vi "Run.vi"(7 "Team Index":i32, 8 "Column":i32, 9 "Row":i32, 10 "View":i32[](array[numeric]) caption="View (Team Index, -1: empty)", 11 "Runner in":refnum<class "Formation.lvclass">) -> (0 "Replicated":refnum<class "Square.lvclass">, 1 "Direction":T1, 2 "Action":T2, 3 "Runner out":refnum<class "Formation.lvclass">)   [LabVIEW 2015, in "Formation.lvclass"]
uses:
  Formation.lvclass
  Type Defs/Action Enum.ctl
  Type Defs/Direction Enum.ctl
  Square/Square.lvclass
  Formation.lvclass/Formation.ctl
  DVR Data Cluster.ctl
  Board Cluster.ctl
  SubVIs/Read-Only Globals.vi
  SubVIs/Globals (private).vi
  Common/Find Enemy.vi
  Common/Reverse Direction.vi
  Type Defs/SB Type Defs.lvlib
  Common/Common.lvlib
panel:
  # "NW\nN\nNE\nE\nSE\nS\nSW\nW"
  # "NOTICE - YOU MUST NOT REMOVE THIS NOTICE. PER THE FOLLOWING LICENSE, YOU MAY REPRODUCE THIS SOFTWARE PROVIDED YOU FOLLOW THE TERMS\nOF THE LICENSE.\n\n---BEGIN BSD LICENSE (http://opensource.org/licenses/BSD-2-Clause)---\nCopyright (c) 2015, Endigit, Inc. <robert@endigit.com>\nAll rights reserved.\n\nRedistribution and use in source and binary forms, with or without modification, are permitted provided that the following conditions are met:\n\n1. Redistributions of source code must retain the above copyright notice, this list of conditions and the following disclaimer.\n\n2. Redistributions in binary form must reproduce the above copyright notice, this list of conditions and the following disclaimer in the documentation and/or other \nmaterials provided with the distribution.\n\nTHIS SOFTWARE IS PROVIDED BY THE COPYRIGHT HOLDERS AND CONTRIBUTORS \"AS IS\" AND ANY EXPRESS OR IMPLIED WARRANTIES, INCLUDING, BUT NOT \nLIMITED TO, THE IMPLIED WARRANTIES OF MERCHANTABILITY AND FITNESS FOR A PARTICULAR PURPOSE ARE DISCLAIMED. IN NO EVENT SHALL THE COPYRIGHT \nHOLDER OR CONTRIBUTORS BE LIABLE FOR ANY DIRECT, INDIRECT, INCIDENTAL, SPECIAL, EXEMPLARY, OR CONSEQUENTIAL DAMAGES (INCLUDING, BUT NOT \nLIMITED TO, PROCUREMENT OF SUBSTITUTE GOODS OR SERVICES; LOSS OF USE, DATA, OR PROFITS; OR BUSINESS INTERRUPTION) HOWEVER CAUSED AND ON \nANY THEORY OF LIABILITY, WHETHER IN CONTRACT, STRICT LIABILITY, OR TORT (INCLUDING NEGLIGENCE OR OTHERWISE) ARISING IN ANY WAY OUT OF THE USE \nOF THIS SOFTWARE, EVEN IF ADVISED OF THE POSSIBILITY OF SUCH DAMAGE.\n---END BSD LICENSE---"
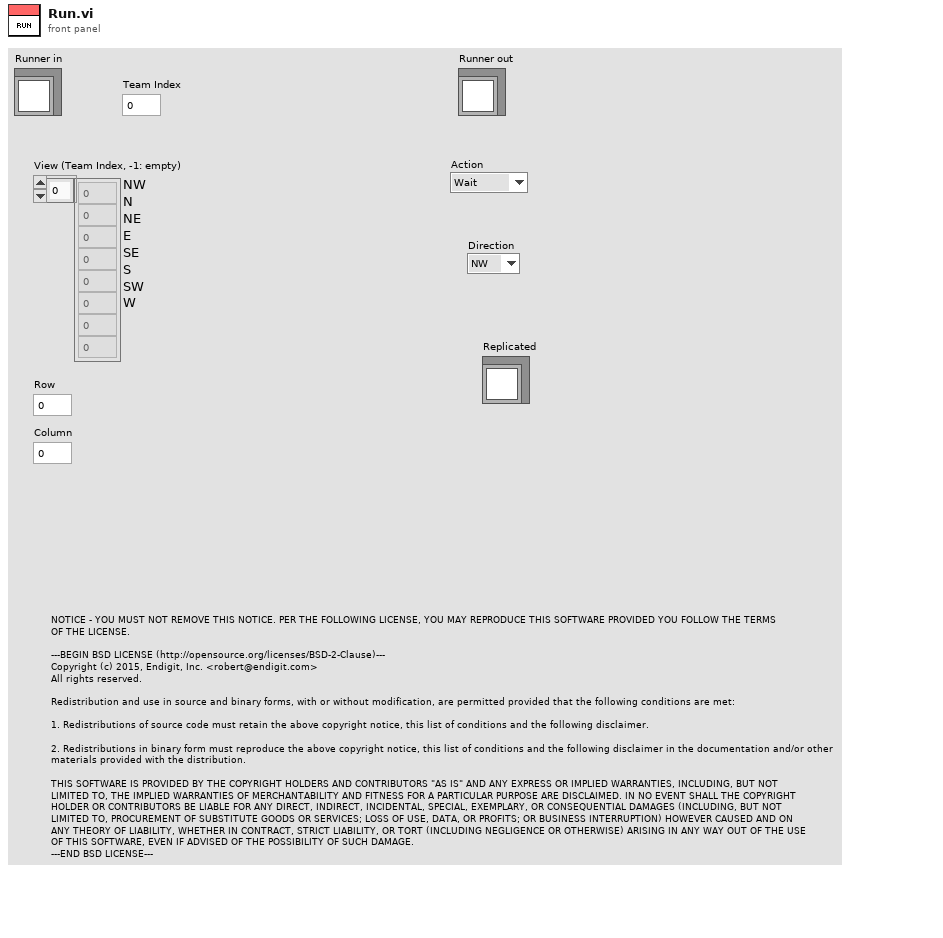
[diagram p1: front panel]
types:
  T1 = typedef "SB Type Defs.lvlib/Direction Enum.ctl" = enum16{"NW", "N", "NE", "E", "SE", "S", "SW", "W"}
  T2 = typedef "SB Type Defs.lvlib/Action Enum.ctl" = enum16{"Wait", "Move", "Attack", "Replicate"}
  T3 = cluster{"Options":cluster{"X":i8, "Y":i8, "SignMatch":i8, "Action":T2, "Direction":T1, "Unit Idx":u8}[]}[]
  T4 = typedef "Formation.lvclass/DVR Data Cluster.ctl" = cluster{"Moved[Id]":i64, "UnitRound":i32, "Direction":T1, "FormIdx":i32, "LastSpawn":i32, "Spawning?":bool, "SpawnDist":i32}
  T5 = cluster{"Options":cluster{"X":i8, "Y":i8, "SignMatch":i8, "Action":T2, "Direction":T1, "Unit Idx":u8}[]}
  T6 = cluster{"X":i8, "Y":i8, "SignMatch":i8, "Action":T2, "Direction":T1, "Unit Idx":u8}[]
  T7 = typedef "Formation.lvclass/Board Cluster.ctl" = cluster{"Board S":i32, "Pos[Idx]":cluster{"X":i32, "Y":i32}[], "Round[Idx]":i32[]}
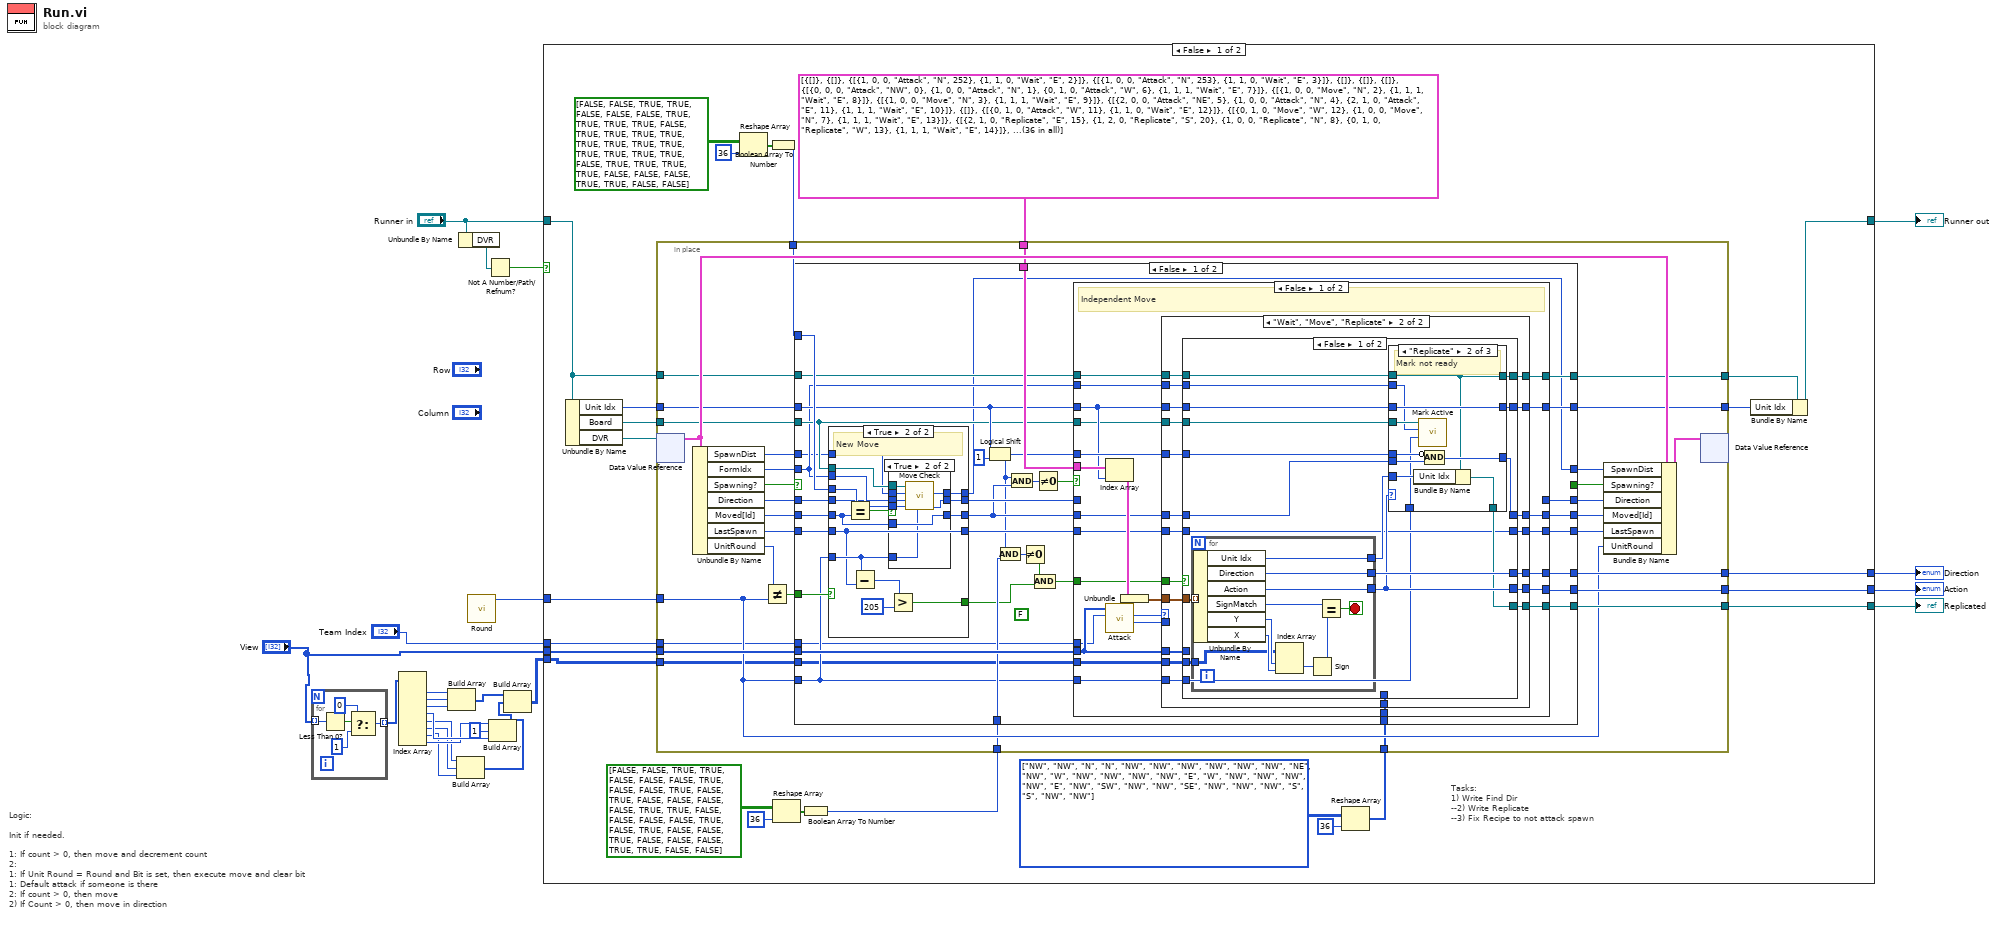
[diagram p0: block diagram]
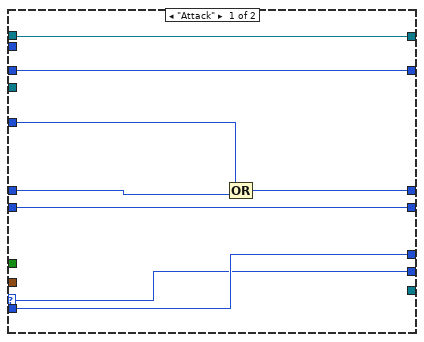
[diagram p2: hidden frame]
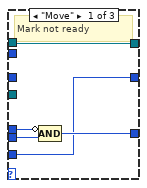
[diagram p3: hidden frame]
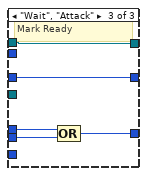
[diagram p4: hidden frame]
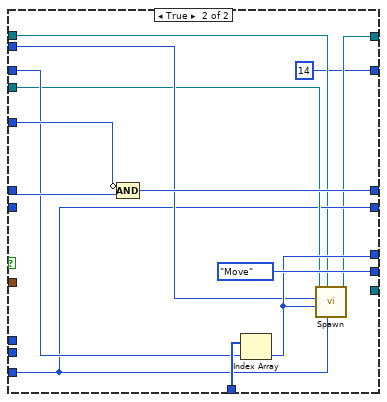
[diagram p5: hidden frame]
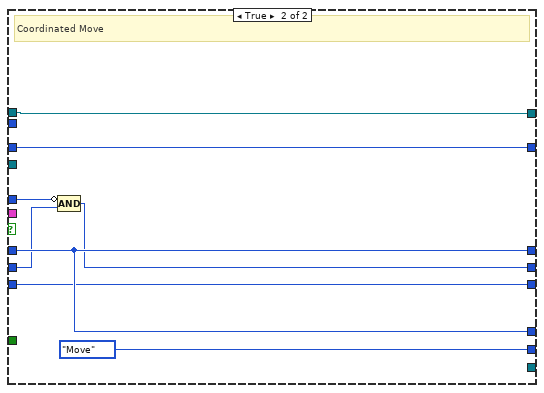
[diagram p6: hidden frame]
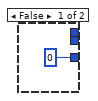
[diagram p8: hidden frame]
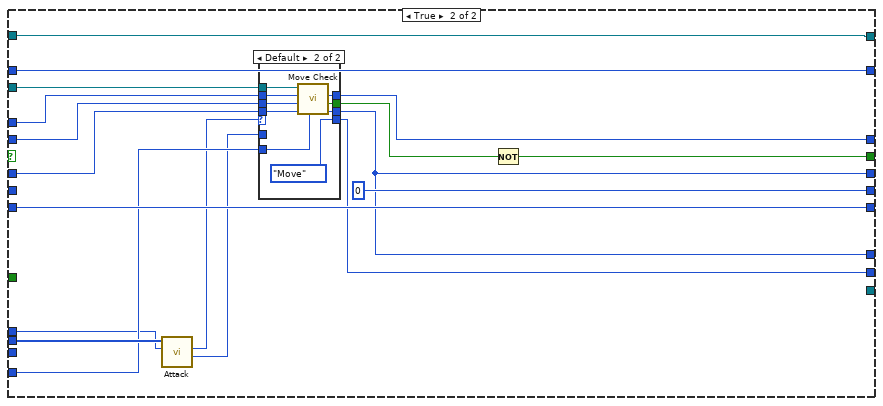
[diagram p9: hidden frame]
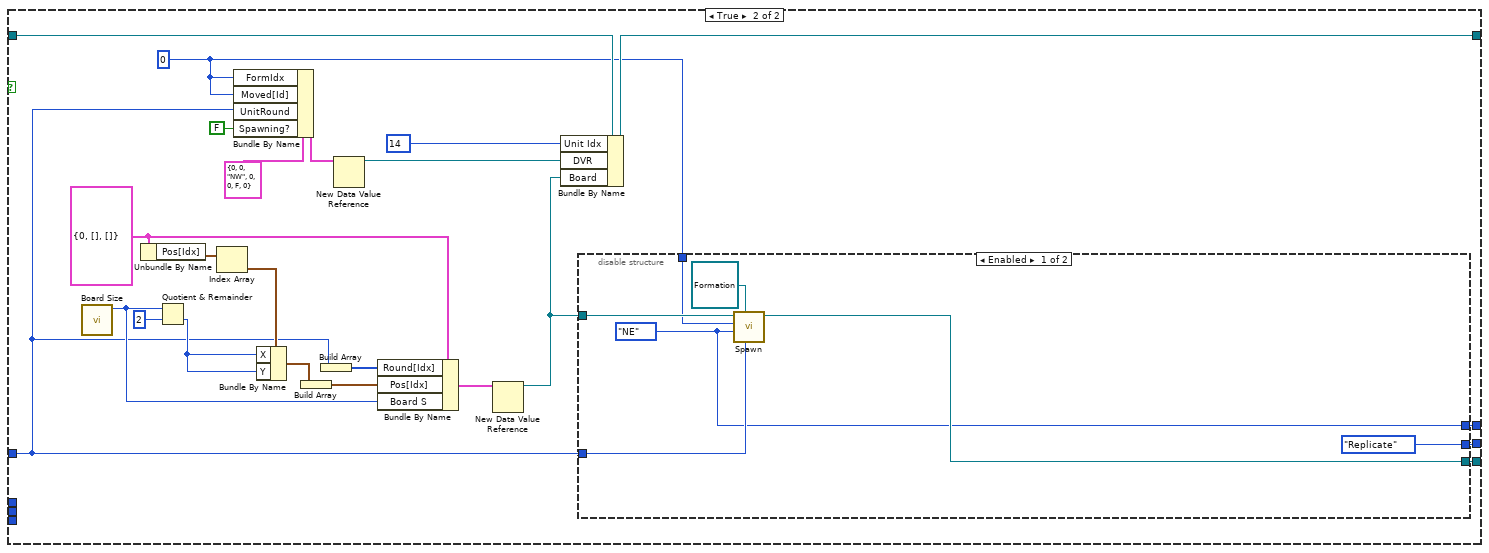
[diagram p11: hidden frame]
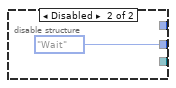
[diagram p12: hidden frame]
diagram:
  # "Logic:\n\nInit if needed.\n\n1: If count > 0, then move and decrement count\n2: \n1: If Unit Round = Round and Bit is set, then execute move and clear bit\n1: Default attack if someone is there\n2: If count > 0, then move\n2) If Count > 0, then move in direction"
  n1 = for {
    tunnel: "View" -> [w29] mode=indexing
    tunnel: [w26] -> w5 mode=indexing
    n2 = Less Than 0?(x=w29) -> (x < 0?=w28:bool)
    n3 = Select(t=0, s=w28, f=1) -> (s? t:f=w26:i32)
  }
  n4 = Index Array(array=w5) -> (element #1=w15:i32, element #2=w14:i32, element #3=w13:i32, element #4=w12:i32, element #5=w9:i32, element #6=w8:i32, element #7=w7:i32, element #8=w11:i32)  [unwired: 8 in]
  n5 = Build Array(w15, w14, w13) -> (w4:i32[])
  n6 = Build Array(w9, w8, w7) -> (w2:i32[])
  n7 = Unbundle By Name("Runner in") -> ("DVR"=w24:refnum<data-value>)
  n8 = call "Round.vi"() -> ("Round"=w23:i32)  [unwired: 11 in]
  n9 = Not A Number/Path/Refnum?(number/path/refnum=w24) -> (NaN/Path/Refnum?=w18:bool)
  n10 = Build Array(w11, 1 ("element"), w12) -> (w3:i32[])
  n11 = Build Array(w4, w3, w2) -> (w1:i32[][])
  n12 = case shown="False" w18 {
    tunnel: w23 -> [w52 w305]
    tunnel: "View" -> [w51 _]
    tunnel: [w50 w304] -> w22
    tunnel: [w49 w319] -> w21
    tunnel: [w44 w321] -> w20
    tunnel: "Runner in" -> [w42 w325]
    tunnel: [w41 w307] -> w19
    tunnel: "Team Index" -> [w31 _]
    tunnel: w1 -> [w30 _]
    frame False {
      w36 = T1[][] [[enum."NW", enum."NW", enum."N", enum."N", enum."NW", enum."NW"], [enum."NW", enum."NW", enum."NW", enum."NW", enum."NE", enum."NW"], [enum."W", enum."NW", enum."NW", enum."NW", enum."NW", enum."E"], [enum."W", enum."NW", enum."NW", enum."NW", enum."NW", enum."E"], [enum."NW", enum."SW", enum."NW", enum."NW", enum."SE", enum."NW"], [enum."NW", enum."NW", enum."S", enum."S", enum."NW", enum."NW"]] items=["NW", "N", "NE", "E", "SE", "S", "SW", "W"]
      # "Tasks: \n1) Write Find Dir\n--2) Write Replicate\n--3) Fix Recipe to not attack spawn"
      n13 = Unbundle By Name(w42) -> ("Unit Idx"=w54:u16, "Board"=w55:refnum<data-value>, "DVR"=w53:refnum<data-value>)
      n14 = Reshape Array(bool[][] [[FALSE, FALSE, TRUE, TRUE, FALSE, FALSE], [FALSE, TRUE, TRUE, TRUE, TRUE, FALSE], [TRUE, TRUE, TRUE, TRUE, TRUE, TRUE], [TRUE, TRUE, TRUE, TRUE, TRUE, TRUE], [FALSE, TRUE, TRUE, TRUE, TRUE, FALSE], [FALSE, FALSE, TRUE, TRUE, FALSE, FALSE]], 36 ("dimension size")) -> (w46:bool[])
      n15 = Boolean Array To Number(Boolean array=w46) -> (number=w45:i64)
      n16 = Reshape Array(bool[][] [[FALSE, FALSE, TRUE, TRUE, FALSE, FALSE], [FALSE, TRUE, FALSE, FALSE, TRUE, FALSE], [TRUE, FALSE, FALSE, FALSE, FALSE, TRUE], [TRUE, FALSE, FALSE, FALSE, FALSE, TRUE], [FALSE, TRUE, FALSE, FALSE, TRUE, FALSE], [FALSE, FALSE, TRUE, TRUE, FALSE, FALSE]], 36 ("dimension size")) -> (w38:bool[])
      n17 = Boolean Array To Number(Boolean array=w38) -> (number=w37:i64)
      n18 = Reshape Array(w36, 36 ("dimension size")) -> (w34:T1[])
      n19 = in-place {
        in-place-border: w54 -> [w75]
        in-place-border: w55 -> [w69]
        in-place-border: w51 -> [w73]
        in-place-border: w52 -> [w67]
        in-place-border: [w80] -> w50
        in-place-border: [w79] -> w49
        in-place-border: w45 -> [w77]
        in-place-border: T3 [{"Options"=[]}, {"Options"=[]}, {"Options"=[{"X"=1, "Y"=0, "SignMatch"=0, "Action"=enum."Attack", "Direction"=enum."N", "Unit Idx"=252}, {"X"=1, "Y"=1, "SignMatch"=0, "Action"=enum."Wait", "Direction"=enum."E", "Unit Idx"=2}]}, {"Options"=[{"X"=1, "Y"=0, "SignMatch"=0, "Action"=enum."Attack", "Direction"=enum."N", "Unit Idx"=253}, {"X"=1, "Y"=1, "SignMatch"=0, "Action"=enum."Wait", "Direction"=enum."E", "Unit Idx"=3}]}, {"Options"=[]}, {"Options"=[]}, {"Options"=[]}, {"Options"=[{"X"=0, "Y"=0, "SignMatch"=0, "Action"=enum."Attack", "Direction"=enum."NW", "Unit Idx"=0}, {"X"=1, "Y"=0, "SignMatch"=0, "Action"=enum."Attack", "Direction"=enum."N", "Unit Idx"=1}, {"X"=0, "Y"=1, "SignMatch"=0, "Action"=enum."Attack", "Direction"=enum."W", "Unit Idx"=6}, {"X"=1, "Y"=1, "SignMatch"=1, "Action"=enum."Wait", "Direction"=enum."E", "Unit Idx"=7}]}, {"Options"=[{"X"=1, "Y"=0, "SignMatch"=0, "Action"=enum."Move", "Direction"=enum."N", "Unit Idx"=2}, {"X"=1, "Y"=1, "SignMatch"=1, "Action"=enum."Wait", "Direction"=enum."E", "Unit Idx"=8}]}, {"Options"=[{"X"=1, "Y"=0, "SignMatch"=0, "Action"=enum."Move", "Direction"=enum."N", "Unit Idx"=3}, {"X"=1, "Y"=1, "SignMatch"=1, "Action"=enum."Wait", "Direction"=enum."E", "Unit Idx"=9}]}, {"Options"=[{"X"=2, "Y"=0, "SignMatch"=0, "Action"=enum."Attack", "Direction"=enum."NE", "Unit Idx"=5}, {"X"=1, "Y"=0, "SignMatch"=0, "Action"=enum."Attack", "Direction"=enum."N", "Unit Idx"=4}, {"X"=2, "Y"=1, "SignMatch"=0, "Action"=enum."Attack", "Direction"=enum."E", "Unit Idx"=11}, {"X"=1, "Y"=1, "SignMatch"=1, "Action"=enum."Wait", "Direction"=enum."E", "Unit Idx"=10}]}, {"Options"=[]}, {"Options"=[{"X"=0, "Y"=1, "SignMatch"=0, "Action"=enum."Attack", "Direction"=enum."W", "Unit Idx"=11}, {"X"=1, "Y"=1, "SignMatch"=0, "Action"=enum."Wait", "Direction"=enum."E", "Unit Idx"=12}]}, {"Options"=[{"X"=0, "Y"=1, "SignMatch"=0, "Action"=enum."Move", "Direction"=enum."W", "Unit Idx"=12}, {"X"=1, "Y"=0, "SignMatch"=0, "Action"=enum."Move", "Direction"=enum."N", "Unit Idx"=7}, {"X"=1, "Y"=1, "SignMatch"=1, "Action"=enum."Wait", "Direction"=enum."E", "Unit Idx"=13}]}, {"Options"=[{"X"=2, "Y"=1, "SignMatch"=0, "Action"=enum."Replicate", "Direction"=enum."E", "Unit Idx"=15}, {"X"=1, "Y"=2, "SignMatch"=0, "Action"=enum."Replicate", "Direction"=enum."S", "Unit Idx"=20}, {"X"=1, "Y"=0, "SignMatch"=0, "Action"=enum."Replicate", "Direction"=enum."N", "Unit Idx"=8}, {"X"=0, "Y"=1, "SignMatch"=0, "Action"=enum."Replicate", "Direction"=enum."W", "Unit Idx"=13}, {"X"=1, "Y"=1, "SignMatch"=1, "Action"=enum."Wait", "Direction"=enum."E", "Unit Idx"=14}]}, {"Options"=[{"X"=1, "Y"=2, "SignMatch"=0, "Action"=enum."Replicate", "Direction"=enum."S", "Unit Idx"=21}, {"X"=1, "Y"=0, "SignMatch"=0, "Action"=enum."Replicate", "Direction"=enum."N", "Unit Idx"=9}, {"X"=2, "Y"=1, "SignMatch"=0, "Action"=enum."Replicate", "Direction"=enum."E", "Unit Idx"=16}, {"X"=1, "Y"=1, "SignMatch"=1, "Action"=enum."Wait", "Direction"=enum."E", "Unit Idx"=15}]}, {"Options"=[{"X"=2, "Y"=1, "SignMatch"=0, "Action"=enum."Move", "Direction"=enum."E", "Unit Idx"=17}, {"X"=1, "Y"=0, "SignMatch"=0, "Action"=enum."Move", "Direction"=enum."N", "Unit Idx"=10}, {"X"=1, "Y"=1, "SignMatch"=1, "Action"=enum."Wait", "Direction"=enum."E", "Unit Idx"=16}]}, {"Options"=[{"X"=2, "Y"=1, "SignMatch"=0, "Action"=enum."Attack", "Direction"=enum."E", "Unit Idx"=18}, {"X"=1, "Y"=1, "SignMatch"=0, "Action"=enum."Wait", "Direction"=enum."E", "Unit Idx"=17}]}, {"Options"=[{"X"=0, "Y"=1, "SignMatch"=0, "Action"=enum."Attack", "Direction"=enum."W", "Unit Idx"=17}, {"X"=1, "Y"=1, "SignMatch"=0, "Action"=enum."Wait", "Direction"=enum."E", "Unit Idx"=18}]}, {"Options"=[{"X"=0, "Y"=1, "SignMatch"=0, "Action"=enum."Move", "Direction"=enum."W", "Unit Idx"=18}, {"X"=1, "Y"=2, "SignMatch"=0, "Action"=enum."Move", "Direction"=enum."S", "Unit Idx"=25}, {"X"=1, "Y"=1, "SignMatch"=1, "Action"=enum."Wait", "Direction"=enum."E", "Unit Idx"=19}]}, {"Options"=[{"X"=1, "Y"=0, "SignMatch"=0, "Action"=enum."Replicate", "Direction"=enum."N", "Unit Idx"=14}, {"X"=1, "Y"=2, "SignMatch"=0, "Action"=enum."Replicate", "Direction"=enum."S", "Unit Idx"=26}, {"X"=0, "Y"=1, "SignMatch"=0, "Action"=enum."Replicate", "Direction"=enum."W", "Unit Idx"=19}, {"X"=1, "Y"=1, "SignMatch"=1, "Action"=enum."Wait", "Direction"=enum."E", "Unit Idx"=20}]}, {"Options"=[{"X"=1, "Y"=0, "SignMatch"=0, "Action"=enum."Replicate", "Direction"=enum."N", "Unit Idx"=15}, {"X"=1, "Y"=2, "SignMatch"=0, "Action"=enum."Replicate", "Direction"=enum."S", "Unit Idx"=27}, {"X"=2, "Y"=1, "SignMatch"=0, "Action"=enum."Replicate", "Direction"=enum."E", "Unit Idx"=22}, {"X"=1, "Y"=1, "SignMatch"=1, "Action"=enum."Wait", "Direction"=enum."E", "Unit Idx"=21}]}, {"Options"=[{"X"=2, "Y"=1, "SignMatch"=0, "Action"=enum."Move", "Direction"=enum."E", "Unit Idx"=23}, {"X"=1, "Y"=2, "SignMatch"=0, "Action"=enum."Move", "Direction"=enum."S", "Unit Idx"=28}, {"X"=1, "Y"=1, "SignMatch"=1, "Action"=enum."Wait", "Direction"=enum."E", "Unit Idx"=22}]}, {"Options"=[{"X"=2, "Y"=1, "SignMatch"=0, "Action"=enum."Attack", "Direction"=enum."E", "Unit Idx"=24}, {"X"=1, "Y"=1, "SignMatch"=0, "Action"=enum."Wait", "Direction"=enum."E", "Unit Idx"=23}]}, {"Options"=[]}, {"Options"=[{"X"=0, "Y"=2, "SignMatch"=0, "Action"=enum."Attack", "Direction"=enum."SW", "Unit Idx"=30}, {"X"=0, "Y"=1, "SignMatch"=0, "Action"=enum."Attack", "Direction"=enum."W", "Unit Idx"=24}, {"X"=1, "Y"=2, "SignMatch"=0, "Action"=enum."Attack", "Direction"=enum."S", "Unit Idx"=31}, {"X"=1, "Y"=1, "SignMatch"=1, "Action"=enum."Wait", "Direction"=enum."E", "Unit Idx"=25}]}, {"Options"=[{"X"=1, "Y"=2, "SignMatch"=0, "Action"=enum."Move", "Direction"=enum."S", "Unit Idx"=32}, {"X"=1, "Y"=1, "SignMatch"=1, "Action"=enum."Wait", "Direction"=enum."E", "Unit Idx"=26}]}, {"Options"=[{"X"=1, "Y"=2, "SignMatch"=0, "Action"=enum."Move", "Direction"=enum."S", "Unit Idx"=33}, {"X"=1, "Y"=1, "SignMatch"=1, "Action"=enum."Wait", "Direction"=enum."E", "Unit Idx"=27}]}, {"Options"=[{"X"=2, "Y"=2, "SignMatch"=0, "Action"=enum."Attack", "Direction"=enum."SE", "Unit Idx"=35}, {"X"=1, "Y"=2, "SignMatch"=0, "Action"=enum."Attack", "Direction"=enum."S", "Unit Idx"=34}, {"X"=2, "Y"=1, "SignMatch"=0, "Action"=enum."Attack", "Direction"=enum."E", "Unit Idx"=29}, {"X"=1, "Y"=1, "SignMatch"=1, "Action"=enum."Wait", "Direction"=enum."E", "Unit Idx"=28}]}, {"Options"=[]}, {"Options"=[]}, {"Options"=[]}, {"Options"=[{"X"=1, "Y"=2, "SignMatch"=0, "Action"=enum."Attack", "Direction"=enum."S", "Unit Idx"=38}, {"X"=1, "Y"=1, "SignMatch"=0, "Action"=enum."Wait", "Direction"=enum."E", "Unit Idx"=32}]}, {"Options"=[{"X"=1, "Y"=2, "SignMatch"=0, "Action"=enum."Attack", "Direction"=enum."S", "Unit Idx"=39}, {"X"=1, "Y"=1, "SignMatch"=0, "Action"=enum."Wait", "Direction"=enum."E", "Unit Idx"=33}]}, {"Options"=[]}, {"Options"=[]}] ("Recipe") -> [w74]
        in-place-border: [w72] -> w43
        in-place-border: w42 -> [w71]
        in-place-border: [w70] -> w41
        in-place-border: w37 -> [w66]
        in-place-border: w34 -> [w64]
        in-place-border: [w60] -> w32
        in-place-border: w31 -> [w57]
        in-place-border: w30 -> [w56]
        n20 = in-place-dvr #1(w53) -> (w85:T4)  [unwired: 1 out]
        n21 = Unbundle By Name(w85) -> ("SpawnDist"=w59:i32, "FormIdx"=w62:i32, "Spawning?"=w63:bool, "Direction"=w61:T1, "Moved[Id]"=w83:i64, "LastSpawn"=w68:i32, "UnitRound"=w76:i32)
        n22 = Not Equal?(x=w76, y=w67) -> (x != y?=w84:bool)
        n23 = case shown="False" w63 {
          tunnel: w84 -> [w123 _]
          tunnel: w83 -> [w122 _]
          tunnel: w61 -> [w121 w285]
          tunnel: [_ w286] -> w82
          tunnel: [w112 w277] -> w81
          tunnel: [w114 w277] -> w80
          tunnel: [w113 w274] -> w79
          tunnel: [w111 i64 0] -> w78
          tunnel: w77 -> [w120 _]
          tunnel: w75 -> [w103 w289]
          tunnel: w74 -> [w110 _]
          tunnel: w73 -> [w109 w279]
          tunnel: [w108 w289] -> w72
          tunnel: w71 -> [w107 w284]
          tunnel: [w106 _] -> w70
          tunnel: w69 -> [w93 w283]
          tunnel: w68 -> [w105 w288]
          tunnel: w67 -> [w95 w278]
          tunnel: w66 -> [w101 _]
          tunnel: [w97 w288] -> w65
          tunnel: w64 -> [w94 _]
          tunnel: w62 -> [w92 w287]
          tunnel: [w91 w284] -> w60
          tunnel: w59 -> [w90 w282]
          tunnel: [w89 w280] -> w58
          tunnel: w57 -> [w88 w273]
          tunnel: w56 -> [w87 _]
          frame False {
            (unwired) FALSE ("value")
            n24 = case shown="True" w123 {
              tunnel: w122 -> [w248 w262]
              tunnel: w121 -> [w247 w251]
              tunnel: w120 -> [_ w263]
              tunnel: [w248 w261] -> w115
              tunnel: [w247 w257] -> w116
              tunnel: w105 -> [w246 w252]
              tunnel: w95 -> [_ w253]
              tunnel: [_ w259] -> w98
              tunnel: [w246 w252] -> w104
              tunnel: w93 -> [_ w258]
              tunnel: w92 -> [_ w256]
              tunnel: w90 -> [_ w250]
              tunnel: [_ w249] -> w89
              frame False {
              }
              frame True {
                # "New Move"
                n25 = Equal?(x=w263, y=w262) -> (x = y?=w254:bool)
                n26 = Subtract(x=w253, y=w252) -> (x-y=w260:i32)
                n27 = case shown="True" w254 {
                  tunnel: w262 -> [_ w271]
                  tunnel: [i64 0 ("f") w271] -> w261
                  tunnel: w258 -> [_ w268]
                  tunnel: [_ w266] -> w257
                  tunnel: w256 -> [_ w272]
                  tunnel: w253 -> [_ w270]
                  tunnel: w251 -> [_ w269]
                  tunnel: w250 -> [_ w267]
                  tunnel: [_ w265] -> w249
                  frame False {
                  }
                  frame True {
                    n28 = call "Move Check.vi"("Round"=w270, "Assumed Dir"=w269, "Idx"=w272, "SpawnDist"=w267, "Board"=w268) -> ("Direction"=w266:T1, "SpawnDist out"=w265:i32)  [unwired: 4 in, 1 out]
                  }
                }
                n29 = Greater?(x=w260, y=205) -> (0:w259:bool)
              }
            }
            n30 = Logical Shift(y=w103, x=i64 1) -> (x << y=w100:i64)
            n31 = And(x=w100, y=w101) -> (x .and. y?=w102:i64)
            n32 = And(x=w100, y=w115) -> (x .and. y?=w118:i64)
            n33 = Not Equal To 0?(x=w102) -> (x != 0?=w99:bool)
            n34 = Not Equal To 0?(x=w118) -> (x != 0?=w117:bool)
            n35 = Compound Arithmetic op=AND(w99, w98) -> (w96:bool)
            n36 = case shown="False" w117 {
              tunnel: w116 -> [_ w244]
              tunnel: w115 -> [w144 w242]
              tunnel: [w145 w244] -> w114
              tunnel: [w143 Action_Enum."Move" ("Action")] -> w113
              tunnel: [_ w244] -> w112
              tunnel: w100 -> [w142 w243]
              tunnel: [w141 w241] -> w111
              tunnel: w110 -> [w148 _]
              tunnel: w103 -> [w138 w240]
              tunnel: w109 -> [w136 _]
              tunnel: [w140 w240] -> w108
              tunnel: w107 -> [w139 w238]
              tunnel: [w137 _] -> w106
              tunnel: w104 -> [w132 w239]
              tunnel: [w131 w239] -> w97
              tunnel: w96 -> [w133 _]
              tunnel: w95 -> [w130 _]
              tunnel: w94 -> [w129 _]
              tunnel: w92 -> [w128 _]
              tunnel: w93 -> [w127 _]
              tunnel: [w126 w238] -> w91
              tunnel: w88 -> [w125 _]
              tunnel: w87 -> [w124 _]
              frame False {
                # "Independent Move"
                n37 = Index Array(array=w148, index=w138) -> (element=w147:T5)
                n38 = call "Attack.vi"("Team Index"=w125, "View"=w136) -> ("Direction"=w134:i32, "Action"=w135:T2)  [unwired: 4 in, 4 out]
                n39 = Unbundle(w147) -> ("Options"=w146:T6)
                n40 = case shown="\"Wait\", \"Move\", \"Replicate\"" w135 {
                  selector: w135 -> [w151 _]
                  tunnel: w146 -> [_ w176]
                  tunnel: [w152 w175] -> w145
                  tunnel: w144 -> [w154 w174]
                  tunnel: [w151 w173] -> w143
                  tunnel: w142 -> [w153 w172]
                  tunnel: [w155 w171] -> w141
                  tunnel: [w156 w170] -> w140
                  tunnel: w139 -> [w149 w169]
                  tunnel: w138 -> [w156 w168]
                  tunnel: [_ w167] -> w137
                  tunnel: w136 -> [_ w166]
                  tunnel: w134 -> [w152 _]
                  tunnel: w133 -> [_ w165]
                  tunnel: w132 -> [w150 w164]
                  tunnel: [w150 w163] -> w131
                  tunnel: w130 -> [_ w162]
                  tunnel: w129 -> [_ w161]
                  tunnel: w128 -> [_ w160]
                  tunnel: w127 -> [_ w159]
                  tunnel: [w149 w158] -> w126
                  tunnel: w124 -> [_ w157]
                  frame "Attack" {
                    n41 = Compound Arithmetic op=OR(w153, w154) -> (w155:i64)
                  }
                  frame "Wait", "Move", "Replicate" {
                    n42 = case shown="False" w165 {
                      tunnel: w176 -> [w193 _]
                      tunnel: [w192 w231] -> w175
                      tunnel: w174 -> [w191 w235]
                      tunnel: [w190 Action_Enum."Move" ("Action")] -> w173
                      tunnel: w172 -> [w189 w234]
                      tunnel: [w188 w236] -> w171
                      tunnel: [w186 u16 14 ("Unit Idx")] -> w170
                      tunnel: w169 -> [w185 w227]
                      tunnel: w168 -> [w184 w232]
                      tunnel: [w183 _] -> w167
                      tunnel: w166 -> [_ _]
                      tunnel: w164 -> [w182 _]
                      tunnel: [w182 w228] -> w163
                      tunnel: w162 -> [w180 w228]
                      tunnel: w161 -> [_ w233]
                      tunnel: w160 -> [w179 w230]
                      tunnel: w159 -> [w181 w229]
                      tunnel: [w178 w226] -> w158
                      tunnel: w157 -> [w177 _]
                      frame False {
                        n43 = for {
                          tunnel: w193 -> [w224] mode=indexing
                          tunnel: [w217] -> w192
                          tunnel: [w216] -> w187
                          tunnel: [w215] -> w190
                          tunnel: w177 -> [w214]
                          stop <- w218 stop-if-true
                          n44 = Unbundle By Name(w224) -> ("Unit Idx"=w216:u8, "Direction"=w217:T1, "Action"=w215:T2, "SignMatch"=w219:i8, "Y"=w223:i8, "X"=w222:i8)
                          n45 = Index Array(array=w214, index (row)=w223, index (col)=w222) -> (element=w221:i32)
                          n46 = Sign(1:w221) -> (0:w220:i32)
                          n47 = Equal?(x=w219, y=w220) -> (x = y?=w218:bool)
                        }
                        n48 = case shown="\"Replicate\"" w190 {
                          tunnel: w191 -> [w198 w208 w213]
                          tunnel: w189 -> [w197 w207 w212]
                          tunnel: [w196 w206 w211] -> w188
                          tunnel: w187 -> [w195 w205 _]
                          tunnel: [w195 w204 w210] -> w186
                          tunnel: w185 -> [w194 w199 w209]
                          tunnel: w184 -> [_ w204 w210]
                          tunnel: [_ w203 _] -> w183
                          tunnel: w181 -> [_ w202 _]
                          tunnel: w180 -> [_ w201 _]
                          tunnel: w179 -> [_ w200 _]
                          tunnel: [w194 w199 w209] -> w178
                          frame "Move" {
                            # "Mark not ready"
                            n49 = Compound Arithmetic op=AND(invert w197, w198) -> (w196:i64)
                          }
                          frame "Replicate" {
                            # "Mark not ready"
                            n50 = Bundle By Name(cluster=w199, "Unit Idx"=w205) -> (w203:refnum<class "Formation.lvclass">)
                            n51 = call "Mark Active.vi"("Round"=w201, "Idx"=w200, "Board"=w202) -> ()  [unwired: 9 in]
                            n52 = Compound Arithmetic op=AND(invert w207, w208) -> (w206:i64)
                          }
                          frame "Wait", "Attack" {
                            # "Mark Ready"
                            n53 = Compound Arithmetic op=OR(w212, w213) -> (w211:i64)
                          }
                        }
                      }
                      frame True {
                        n54 = Compound Arithmetic op=AND(invert w234, w235) -> (w236:i64)
                        n55 = Index Array(array=w233, index=w232) -> (element=w231:T1)
                        n56 = call "Spawn.vi"("Round"=w228, "Runner in"=w227, "Direction"=w231, "Parent Idx"=w230, "Board"=w229) -> ("Replicated"=w226:refnum<class "Formation.lvclass">)  [unwired: 6 in]
                      }
                    }
                  }
                }
              }
              frame True {
                # "Coordinated Move"
                n57 = Compound Arithmetic op=AND(invert w243, w242) -> (w241:i64)
              }
            }
          }
          frame True {
            n58 = call "Attack.vi"("Team Index"=w273, "View"=w279) -> ("Direction"=w275:i32, "Action"=w276:T2)  [unwired: 4 in, 4 out]
            n59 = case shown="Default" w276 {
              selector: w276 -> [w291 _]
              tunnel: w287 -> [_ w302]
              tunnel: w285 -> [_ w301]
              tunnel: w283 -> [_ w300]
              tunnel: w282 -> [w293 w299]
              tunnel: [_ w298] -> w281
              tunnel: [w293 w297] -> w280
              tunnel: [w292 w296] -> w277
              tunnel: w278 -> [_ w295]
              tunnel: w275 -> [w292 _]
              tunnel: [w291 Action_Enum."Move" ("Action")] -> w274
              frame "Attack" {
              }
              frame Default {
                n60 = call "Move Check.vi"("Round"=w295, "Assumed Dir"=w301, "Idx"=w302, "SpawnDist"=w299, "Board"=w300) -> ("Direction"=w296:T1, "Spawn Can End?"=w298:bool, "SpawnDist out"=w297:i32)  [unwired: 4 in]
              }
            }
            n61 = Not(x=w281) -> (.not. x?=w286:bool)
          }
        }
        n62 = Bundle By Name(cluster=w85, "SpawnDist"=w58, "Spawning?"=w82, "Direction"=w81, "Moved[Id]"=w78, "LastSpawn"=w65, "UnitRound"=w67) -> (w86:T4)
        n63 = in-place-dvr #1(w86) -> ()  [unwired: 2 out]
      }
      n64 = Bundle By Name(cluster=w32, "Unit Idx"=w43) -> (w44:refnum<class "Formation.lvclass">)
    }
    frame True {
      w316 = T7 {"Board S"=0, "Pos[Idx]"=[], "Round[Idx]"=[]} ("Cluster")
      w306 = i64 0 ("Moved[Id]")
      n65 = call "Board Size.vi"() -> ("Board Size"=w317:i32)  [unwired: 11 in]
      n66 = Unbundle By Name(w316) -> ("Pos[Idx]"=w315:cluster{"X":i32, "Y":i32}[])
      n67 = Quotient & Remainder(x=w317, y=2) -> (floor(x/y)=w313:i32)  [unwired: 1 out]
      n68 = Index Array(array=w315) -> (element=w314:cluster{"X":i32, "Y":i32})  [unwired: 1 in]
      n69 = Bundle By Name(cluster=T4 {"Moved[Id]"=0, "UnitRound"=0, "Direction"=enum."NW", "FormIdx"=0, "LastSpawn"=0, "Spawning?"=FALSE, "SpawnDist"=0} ("Cluster"), "FormIdx"=w306, "Moved[Id]"=w306, "UnitRound"=w305, "Spawning?"=FALSE) -> (w320:T4)
      n70 = Bundle By Name(cluster=w314, "X"=w313, "Y"=w313) -> (w312:cluster{"X":i32, "Y":i32})
      n71 = Build Array(w312) -> (w311:cluster{"X":i32, "Y":i32}[])
      n72 = Build Array(w305) -> (w310:i32[])
      n73 = New Data Value Reference(data value=w320) -> (data value reference=w323:refnum<data-value>)  [unwired: 1 in, 1 out]
      n74 = Bundle By Name(cluster=w316, "Round[Idx]"=w310, "Pos[Idx]"=w311, "Board S"=w317) -> (w309:T7)
      n75 = New Data Value Reference(data value=w309) -> (data value reference=w303:refnum<data-value>)  [unwired: 1 in, 1 out]
      n76 = Bundle By Name(cluster=w325, "Unit Idx"=u16 14, "DVR"=w323, "Board"=w303) -> (w321:refnum<class "Formation.lvclass">)
      n77 = disable-structure shown="Enabled" {
        disable-tunnel: [Action_Enum."Replicate" ("Action") Action_Enum."Wait" ("Action")] -> w319
        disable-tunnel: w303 -> [w331 _]
        disable-tunnel: [w330 _] -> w307
        disable-tunnel: w306 -> [w329 _]
        disable-tunnel: w305 -> [w328 _]
        disable-tunnel: [w327 _] -> w304
        frame Enabled {
          w327 = Direction_Enum."NE" ("Direction")
          n78 = call "Spawn.vi"("Round"=w328, "Runner in"=refnum<class "Formation.lvclass"> refnum, "Direction"=w327, "Parent Idx"=w329, "Board"=w331) -> ("Replicated"=w330:refnum<class "Formation.lvclass">)  [unwired: 6 in]
        }
        frame Disabled {
        }
      }
    }
  }
  "Runner out" <- w20
  "Action" <- w21
  "Direction" <- w22
  "Replicated" <- w19
